vi "CRYClear Main Receiver Array.vi"(9 "isMain":bool, 11 "Rcv Idx":i32) -> ()   [LabVIEW 2013]
uses:
  CRYMisc vis settings global.vi
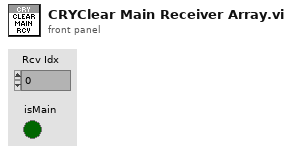
[diagram p1: front panel]
types:
  T1 = cluster{"Rcv Idx":i32, "Chn Idx":i32, "Data":i32[], "bufCount":i32}[]
  T2 = cluster{"Rcv Idx":i32, "Chn Idx":i32, "Data":i32[], "bufCount":i32}
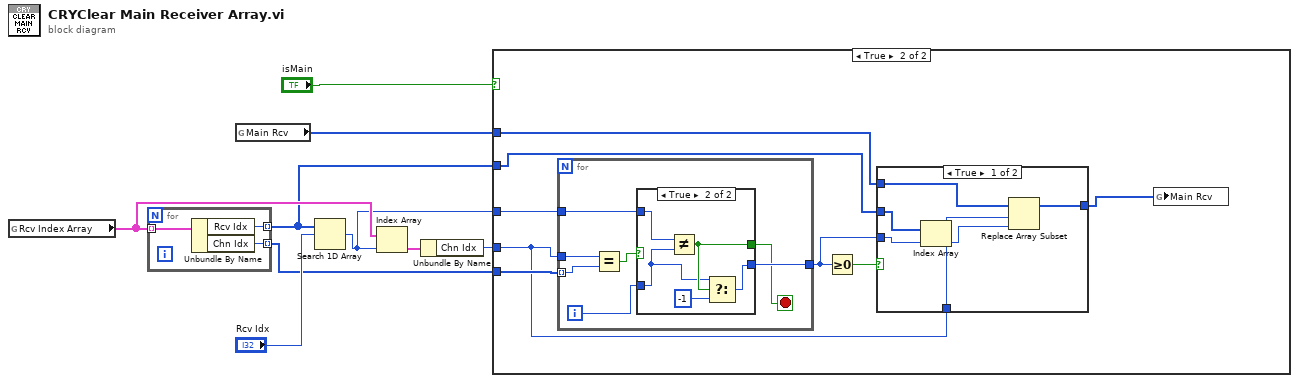
[diagram p0: block diagram]
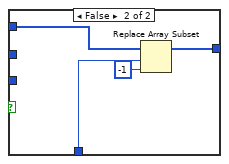
[diagram p3: hidden frame]
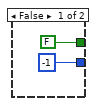
[diagram p4: hidden frame]
diagram:
  n1 = global read "CRYMisc vis settings global.vi" "Rcv Index Array"() -> (w8:T1)
  n2 = for {
    tunnel: w8 -> [w12] mode=indexing
    tunnel: [w11] -> w4 mode=indexing
    tunnel: [w10] -> w3 mode=indexing
    n3 = Unbundle By Name(w12) -> ("Rcv Idx"=w11:i32, "Chn Idx"=w10:i32)
  }
  n4 = global read "CRYMisc vis settings global.vi" "Main Rcv"() -> (w1:i32[])
  n5 = Search 1D Array(1D array=w4, element="Rcv Idx") -> (index of element=w2:i32)  [unwired: 1 in]
  n6 = Index Array(array=w8, index=w2) -> (element=w7:T2)
  n7 = Unbundle By Name(w7) -> ("Chn Idx"=w5:i32)
  n8 = case shown="True" "isMain" {
    tunnel: w5 -> [_ w14]
    tunnel: w4 -> [_ w18]
    tunnel: w3 -> [_ w20]
    tunnel: w2 -> [_ w19]
    tunnel: w1 -> [_ w16]
    frame False {
    }
    frame True {
      n9 = for {
        tunnel: w20 -> [w35] mode=indexing
        tunnel: w14 -> [w37]
        tunnel: w19 -> [w33]
        tunnel: [w32] -> w15
        i -> [w34]
        stop <- w31 stop-if-true
        n10 = Equal?(x=w37, y=w35) -> (x = y?=w36:bool)
        n11 = case shown="True" w36 {
          tunnel: w34 -> [_ w42]
          tunnel: w33 -> [_ w44]
          tunnel: [FALSE w43] -> w31
          tunnel: [-1 w40] -> w32
          frame False {
          }
          frame True {
            n12 = Not Equal?(x=w44, y=w42) -> (x != y?=w43:bool)
            n13 = Select(t=w42, s=w43, f=-1) -> (s? t:f=w40:i32)
          }
        }
      }
      n14 = Greater Or Equal To 0?(x=w15) -> (x >= 0?=w17:bool)
      n15 = case shown="True" w17 {
        tunnel: w18 -> [w26 _]
        tunnel: w16 -> [w24 w30]
        tunnel: w15 -> [w25 _]
        tunnel: w14 -> [w22 w29]
        tunnel: [w21 w28] -> w13
        frame True {
          n16 = Index Array(array=w26, index=w25) -> (element=w23:i32)
          n17 = Replace Array Subset(array=w24, new element=w23, index=w22) -> (w21:i32[])
        }
        frame False {
          n18 = Replace Array Subset(array=w30, new element=-1 ("new element/subarray"), index=w29) -> (w28:i32[])
        }
      }
      n19 = global write "CRYMisc vis settings global.vi" "Main Rcv"(w13) -> ()
    }
  }
